vi "__FilterSet_Submit.vi"(0 "Param in":cluster{"mode":u8, "AccCode":u32, "AccMask":u32}, 5 "CtrlRef":T1, 7 "IDRef":refnum<vi>[](array[refnum]), 9 "EIDRef":refnum<vi>[](array[refnum]), 11 "error in (no error)":errorcluster, 12 "IDRef 2":refnum<vi>[](array[refnum]), 13 "EIDRef 2":refnum<vi>[](array[refnum])) -> (4 "Param out":cluster{"mode":u8, "AccCode":u32, "AccMask":u32}, 15 "error out":errorcluster)   [LabVIEW 2011]
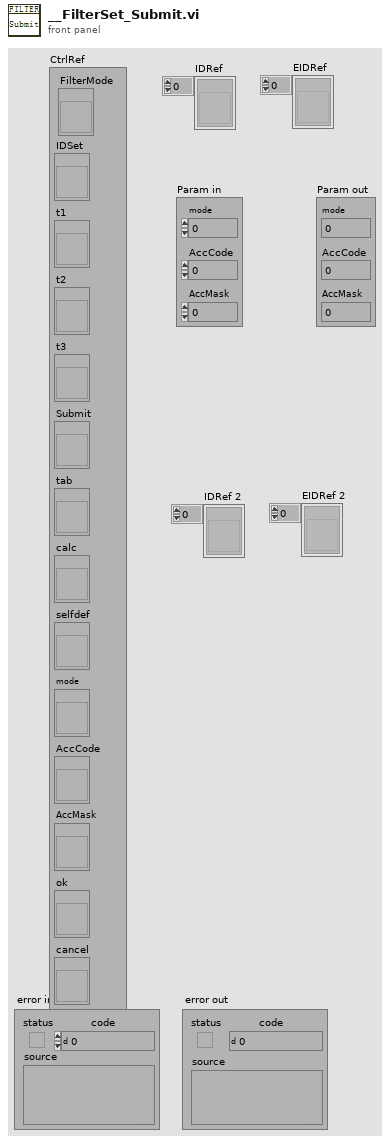
[diagram p1: front panel]
types:
  T1 = cluster{"FilterMode":refnum<vi>, "IDSet":refnum<vi>, "t1":refnum<vi>, "t2":refnum<vi>, "t3":refnum<vi>, "Submit":refnum<vi>, "tab":refnum<vi>, "calc":refnum<vi>, "selfdef":refnum<vi>, "mode":refnum<vi>, "AccCode":refnum<vi>, "AccMask":refnum<vi>, "ok":refnum<vi>, "cancel":refnum<vi>}
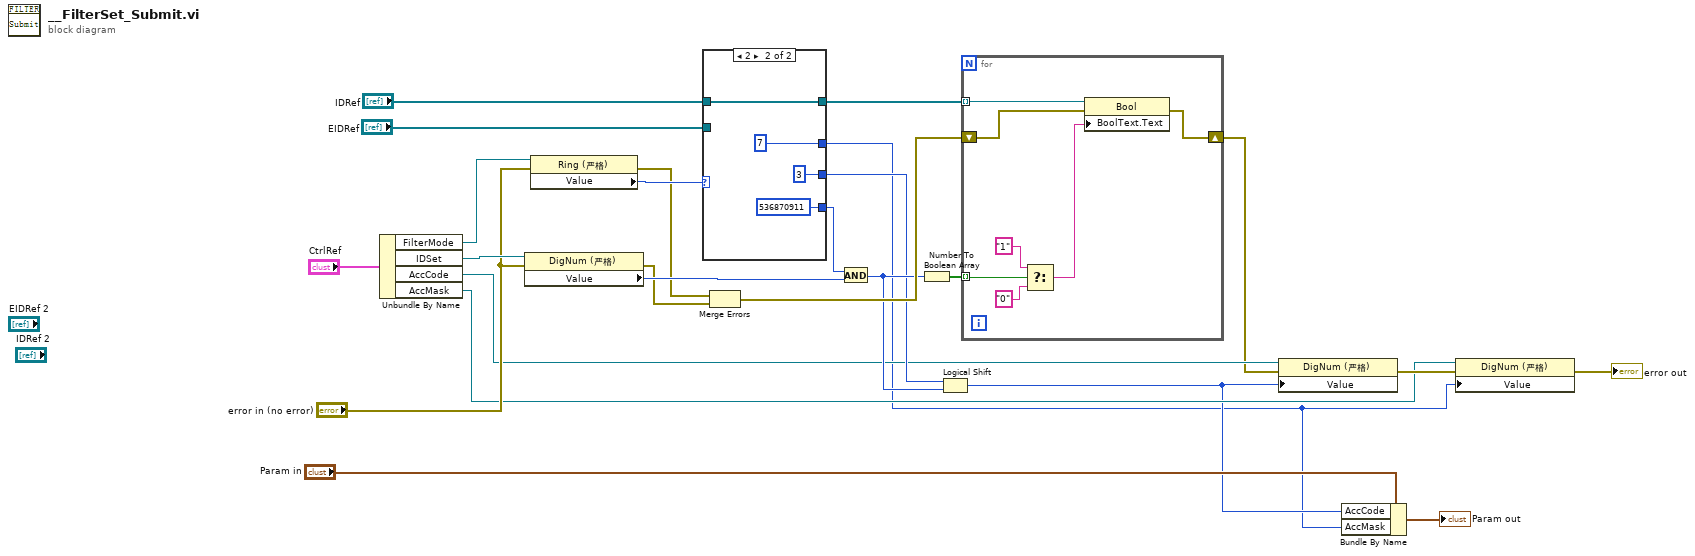
[diagram p0: block diagram]
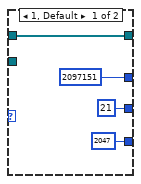
[diagram p2: hidden frame]
diagram:
  n1 = Unbundle By Name("CtrlRef") -> ("FilterMode"=w25:refnum<vi>, "IDSet"=w24:refnum<vi>, "AccCode"=w10:refnum<vi>, "AccMask"=w7:refnum<vi>)
  n2 = property class="DigNum (严格)"(reference=w24, error in="error in (no error)") -> (error out=w14:errorcluster, "Value"=w19:u32)  [unwired: 1 out]
  n3 = property class="Ring (严格)"(reference=w25, error in="error in (no error)") -> (error out=w15:errorcluster, "Value"=w22:u16)  [unwired: 1 out]
  n4 = case shown="2" w22 {
    tunnel: "IDRef" -> [w28 _]
    tunnel: "EIDRef" -> [_ w32]
    tunnel: [u32 2047 u32 536870911] -> w18
    tunnel: [w28 w32] -> w17
    tunnel: [21 3] -> w11
    tunnel: [u32 2097151 u32 7] -> w2
    frame 1, Default {
    }
    frame 2 {
    }
  }
  n5 = Merge Errors(w15, w14) -> (w13:errorcluster)
  n6 = And(x=w18, y=w19) -> (x .and. y?=w12:u32)
  n7 = Number To Boolean Array(number=w12) -> (Boolean array=w16:bool[])
  n8 = Logical Shift(y=w11, x=w12) -> (x << y=w3:u32)
  n9 = for {
    tunnel: w17 -> [w40] mode=indexing
    tunnel: w16 -> [w37] mode=indexing
    shift-right: [w38] -> w9
    shift-left: w13 -> [w39]
    n10 = Select(t="1", s=w37, f="0") -> (s? t:f=w34:string)
    n11 = property class="Bool"(reference=w40, error in=w39, "BoolText.Text"=w34) -> (error out=w38:errorcluster)  [unwired: 1 out]
  }
  n12 = property class="DigNum (严格)"(reference=w10, error in=w9, "Value"=w3) -> (error out=w8:errorcluster)  [unwired: 1 out]
  n13 = Bundle By Name(cluster="Param in", "AccCode"=w3, "AccMask"=w2) -> (→"Param out":cluster{"mode":u8, "AccCode":u32, "AccMask":u32})
  n14 = property class="DigNum (严格)"(reference=w7, error in=w8, "Value"=w2) -> (error out=→"error out":errorcluster)  [unwired: 1 out]
